vi "Global 1.vi"() -> ()   [LabVIEW 2017]
panel:
  out "RESET FOR PRINT":bool
  out "BOM ALARM LAST2 ST 5":bool
  out "BOM ALARM LAST ST 5":bool
  out "BOM ALARM LAST2 ST 4":bool
  out "BOM ALARM LAST ST 4":bool
  out "BOM ALARM LAST2 ST 3":bool
  out "BOM ALARM LAST ST 3":bool
  out "BOM ALARM LAST2 ST 2":bool
  out "BOM ALARM LAST ST 2":bool
  out "PLC COMM":bool
  out "BOM ALARM LAST2 ST 1":bool
  out "BOM ALARM LAST ST 1":bool
  out "CYCLE START 6":bool
  out "CYCLE START 5":bool
  out "CYCLE START 4":bool
  out "CYCLE START 3":bool
  out "CYCLE START 2":bool
  out "CYCLE START 1":bool
  in  "result6":bool
  in  "result5":bool
  in  "result4":bool
  in  "result3":bool
  in  "result2":bool
  in  "result1":bool
  in  "scanner 6":string
  in  "scanner 5":string
  in  "scanner 4":string
  in  "scanner 3":string
  in  "scanner 2":string
  in  "scanner 1":string
  in  "RECIPE NAME":string
  out "MODEL SELECTION":bool
  out "REMOVE VI":bool
  out "REMOVE VI SUBPANEL SETTING":bool
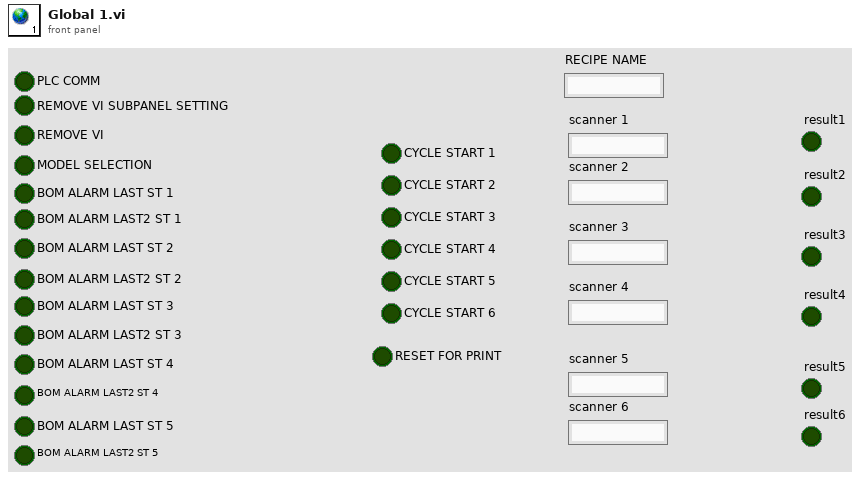
[diagram p1: front panel]
diagram:
